vi "autoshutdown.vi"   [LabVIEW 2016]
uses:
  Instrument_Setup.vi
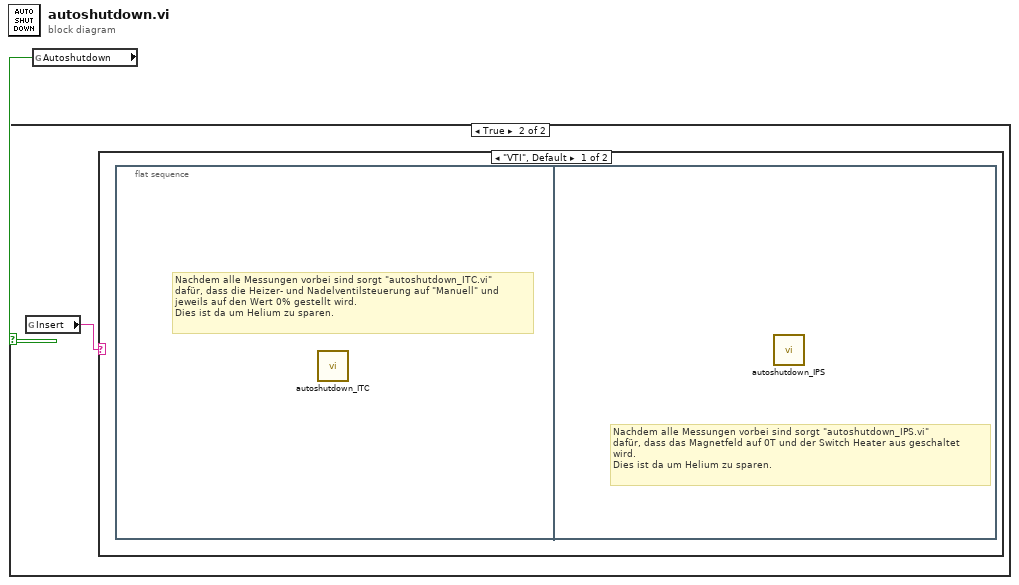
[diagram p0: block diagram]
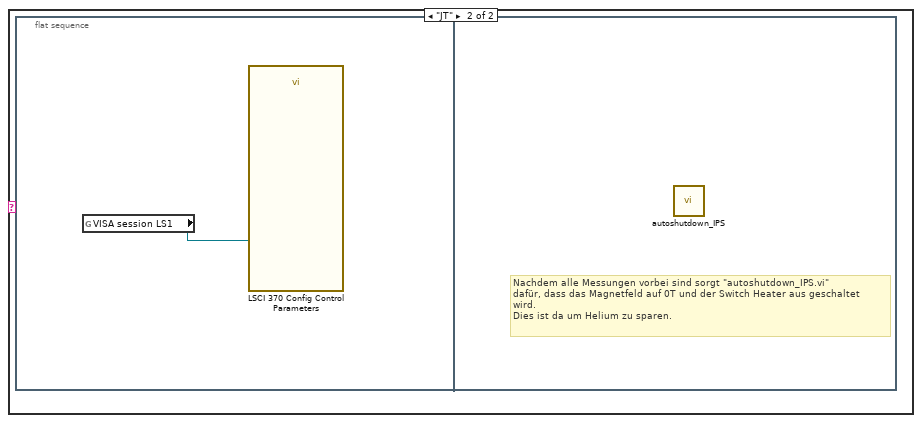
[diagram p3: hidden frame]
diagram:
  n1 = global read "Instrument_Setup.vi" "Autoshutdown"() -> (w1:bool)
  n2 = case shown="True" w1 {
    frame False {
    }
    frame True {
      n3 = global read "Instrument_Setup.vi" "Insert"() -> (w2:string)
      n4 = case shown="\"VTI\", Default" w2 {
        frame "VTI", Default {
          n5 = flat-sequence {
            frame #0 {
              # "Nachdem alle Messungen vorbei sind sorgt \"autoshutdown_ITC.vi\"\ndafür, dass die Heizer- und Nadelventilsteuerung auf \"Manuell\" und\njeweils auf den Wert 0% gestellt wird.\nDies ist da um Helium zu sparen."
              n6 = call "autoshutdown_ITC.vi"() -> ()  [unwired: 1 in]
            }
            frame #1 {
              # "Nachdem alle Messungen vorbei sind sorgt \"autoshutdown_IPS.vi\"\ndafür, dass das Magnetfeld auf 0T und der Switch Heater aus geschaltet\nwird.\nDies ist da um Helium zu sparen."
              n7 = call "autoshutdown_IPS.vi"() -> ()  [unwired: 1 in]
            }
          }
        }
        frame "JT" {
          n8 = flat-sequence {
            frame #0 {
              n9 = global read "Instrument_Setup.vi" "VISA session LS1"() -> (w3:refnum<visa-resource-name>)
              n10 = call "LSCI 370 Config Control Parameters.vi"("VISA session"=w3) -> ()  [unwired: 13 in, 2 out]
            }
            frame #1 {
              # "Nachdem alle Messungen vorbei sind sorgt \"autoshutdown_IPS.vi\"\ndafür, dass das Magnetfeld auf 0T und der Switch Heater aus geschaltet\nwird.\nDies ist da um Helium zu sparen."
              n11 = call "autoshutdown_IPS.vi"() -> ()  [unwired: 1 in]
            }
          }
        }
      }
    }
  }
